vi "Enable Populated Slots Vacuum.vi"(8 "error in":errorcluster, 11 "Gantry in":refnum<class "Gantry Class.lvclass">) -> (0 "error out":errorcluster, 3 "Gantry out":refnum<class "Gantry Class.lvclass">)   [LabVIEW 2017, in "Gantry Class.lvclass"]
uses:
  Gantry Class.lvclass
  WorkTable Class/WorkTable Class.lvclass
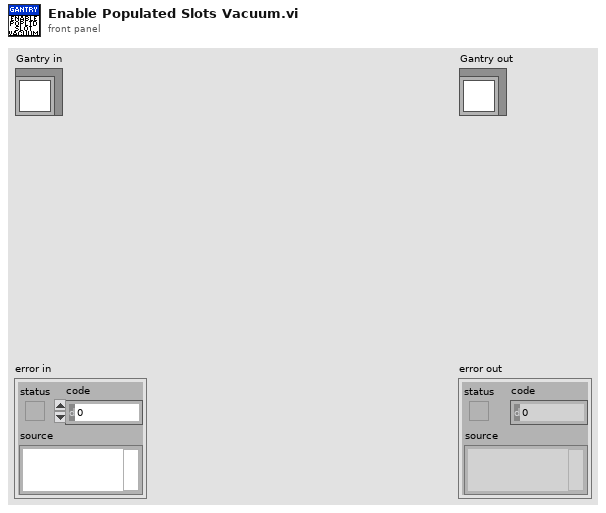
[diagram p1: front panel]
types:
  T1 = enum16{"Empty", "Unglued", "Stamped", "PartOnTop", "Weighted", "Unpotted", "Potted"}
  T2 = typedef "Worktable_Module Slot.ctl" = cluster{"Slot State":enum16{"Empty", "Bare HDI", "Unglued", "Stamped", "PartOnTop", "Weighted", "Unpotted", "Potted"}, "BBM Type":enum16{"None", "BBM", "GlassSlide"}, "HDI Type":enum16{"None", "HDI", "Polyimide"}, "Vacuum Channel":u8, "Location/Orientation BBM":T3, "Location/Orientation HDI":T3, "S/N":string}
  T3 = typedef "Position_Orientation.ctl" = cluster{"Center":refnum<class "Vec3d Class.lvclass">, "Orientation":refnum<class "Orient3d Class.lvclass">}
  T4 = enum16{"Empty", "Bare HDI", "Unglued", "Stamped", "PartOnTop", "Weighted", "Unpotted", "Potted"}
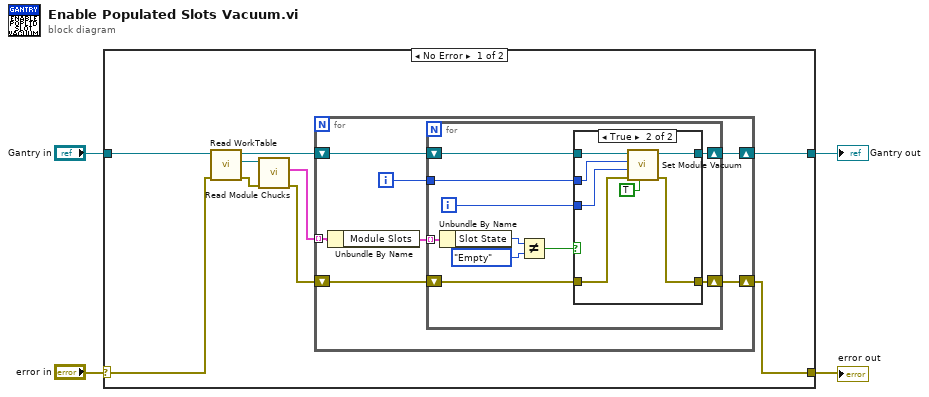
[diagram p0: block diagram]
diagram:
  n1 = case shown="No Error" "error in" {
    selector: "error in" -> [w13 w41]
    tunnel: [w7 w41] -> w2
    tunnel: "Gantry in" -> [w6 w40]
    tunnel: [w5 w40] -> w1
    frame No Error {
      n2 = call-dynamic "Read WorkTable.vi"("error in"=w13, "Gantry Class in"=w6) -> ("error out"=w9:errorcluster, "WorkTable Class.lvclass"=w12:refnum<class "WorkTable Class.lvclass">, "Gantry Class out"=w10:refnum<class "Gantry Class.lvclass">)  [unwired: 7 in]
      n3 = call-dynamic "Read Module Chucks.vi"("error in"=w9, "WorkTable in"=w12) -> ("error out"=w8:errorcluster, "Module Chucks"=w11:cluster{"Module Slots":T2[]}[])  [unwired: 7 in, 1 out]
      n4 = for {
        tunnel: w11 -> [w20] mode=indexing
        shift-right: [w17] -> w5
        shift-left: w10 -> [w18]
        shift-right: [w14] -> w7
        shift-left: w8 -> [w15]
        i -> [w16]
        n5 = Unbundle By Name(w20) -> ("Module Slots"=w19:T2[])
        n6 = for {
          tunnel: w19 -> [w30] mode=indexing
          shift-right: [w25] -> w17
          shift-left: w18 -> [w26]
          tunnel: w16 -> [w24]
          shift-right: [w21] -> w14
          shift-left: w15 -> [w22]
          i -> [w23]
          n7 = Unbundle By Name(w30) -> ("Slot State"=w29:T4)
          n8 = Not Equal?(x=w29, y=T1."Empty") -> (x != y?=w27:bool)
          n9 = case shown="True" w27 {
            tunnel: w26 -> [w32 w39]
            tunnel: [w32 w38] -> w25
            tunnel: w24 -> [_ w36]
            tunnel: w23 -> [_ w35]
            tunnel: w22 -> [w31 w34]
            tunnel: [w31 w33] -> w21
            frame False {
            }
            frame True {
              n10 = call-dynamic "Set Module Vacuum.vi"("On/Off"=TRUE, "error in"=w34, "Slot Number"=w35, "Chuck Number"=w36, "Gantry in"=w39) -> ("error out"=w33:errorcluster, "Gantry out"=w38:refnum<class "Gantry Class.lvclass">)  [unwired: 5 in]
            }
          }
        }
      }
    }
    frame Error {
    }
  }
  "error out" <- w2
  "Gantry out" <- w1
